vi "Restart Alarm Message.vi"(0 "Location":string, 1 "CMD Starts:":i32[](array[numeric]), 2 "Restarts:":i32[](array[numeric]), 3 "High Limits:":i32[](array[numeric]), 4 "Low Limits:":i32[](array[numeric]), 5 "Cog Events":i32[](array[numeric]), 7 "Cog Limits:":i32[](array[numeric])) -> (14 "Subject:":string, 15 "Message:":string)   [LabVIEW 2019]
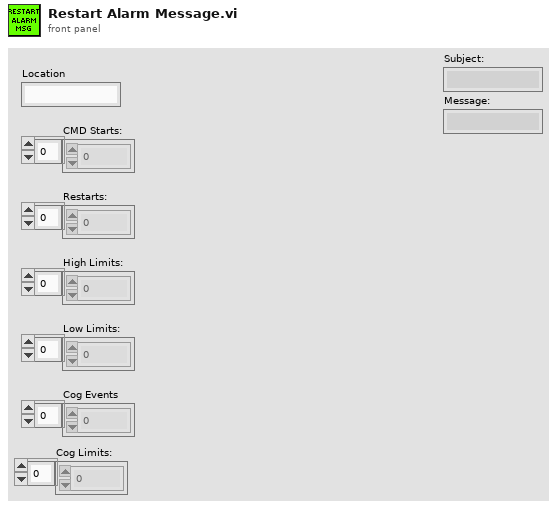
[diagram p1: front panel]
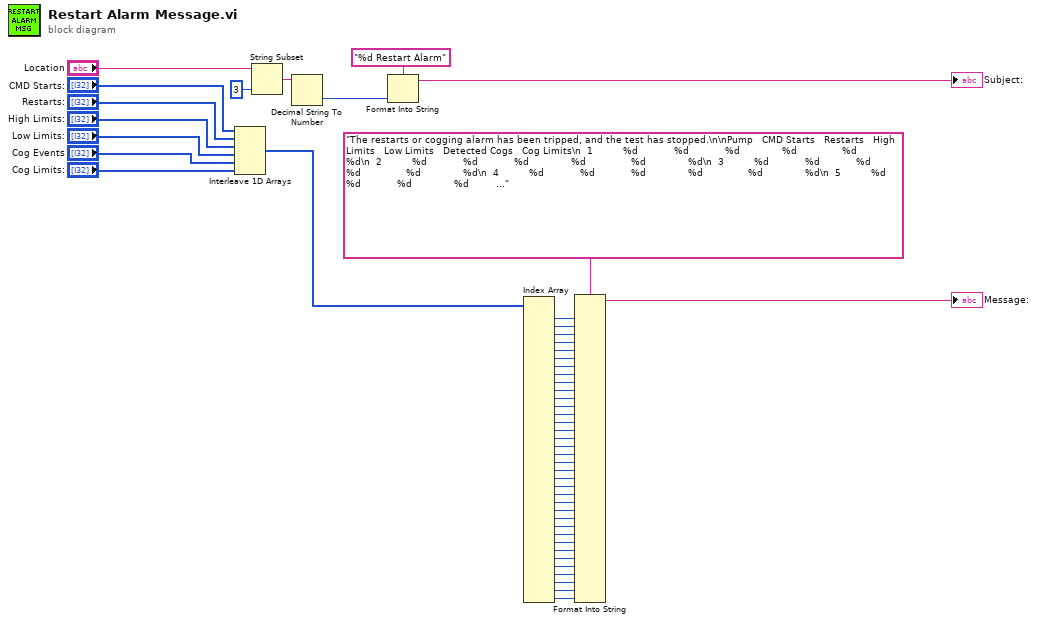
[diagram p0: block diagram]
diagram:
  n1 = Interleave 1D Arrays("CMD Starts:", "Restarts:", "High Limits:", "Low Limits:", "Cog Events", "Cog Limits:") -> (w2:i32[])
  n2 = String Subset(string="Location", length (rest)=3 ("length (rest)")) -> (substring=w51:string)  [unwired: 1 in]
  n3 = Decimal String To Number(string=w51) -> (number=w41:i32)  [unwired: 2 in, 1 out]
  n4 = Format Into String(format string="%d Restart Alarm", w41) -> (resulting string=→"Subject:":string)  [unwired: 2 in, 1 out]
  n5 = Index Array(array=w2) -> (element #1=w26:i32, element #2=w25:i32, element #3=w24:i32, element #4=w23:i32, element #5=w22:i32, element #6=w21:i32, element #7=w20:i32, element #8=w19:i32, element #9=w18:i32, element #10=w17:i32, element #11=w16:i32, element #12=w15:i32, element #13=w13:i32, element #14=w14:i32, element #15=w12:i32, element #16=w11:i32, element #17=w10:i32, element #18=w9:i32, element #19=w8:i32, element #20=w7:i32, element #21=w6:i32, element #22=w5:i32, element #23=w4:i32, element #24=w3:i32, element #25=w28:i32, element #26=w29:i32, element #27=w30:i32, element #28=w31:i32, element #29=w32:i32, element #30=w33:i32, element #31=w34:i32, element #32=w35:i32, element #33=w36:i32, element #34=w37:i32, element #35=w38:i32, element #36=w39:i32)  [unwired: 36 in]
  n6 = Format Into String(format string="The restarts or cogging alarm has been tripped, and the test has stopped.\n\nPump   CMD Starts   Restarts   High Limits   Low Limits   Detected Cogs   Cog Limits\n  1          %d            %d            %d              %d               %d              %d\n  2          %d            %d            %d              %d               %d              %d\n  3          %d            %d            %d              %d               %d              %d\n  4          %d            %d            %d              %d               %d              %d\n  5          %d            %d            %d              %d               %d              %d\n  6          %d            %d            %d              %d               %d              %d" ("Message"), w26, w25, w24, w23, w22, w21, w20, w19, w18, w17, w16, w15, w13, w14, w12, w11, w10, w9, w8, w7, w6, w5, w4, w3, w28, w29, w30, w31, w32, w33, w34, w35, w36, w37, w38, w39) -> (resulting string=→"Message:":string)  [unwired: 2 in, 1 out]
